vi "Send P2P FIFO to AI Loop.vi"(0 "SendDebugVal":bool, 3 "DebugVals":u32, 4 "NoOfSamples":u16, 5 "LastIterration":bool, 6 "SensorID":u8, 7 "FirstIterration":bool, 8 "ActiveLedIndex":u16, 9 "SendAiTrig":u16, 10 "SendAiCMD":u16, 11 "TimingCounter":u16) -> (1 "Trig":bool, 2 "Timed Out?":bool)   [LabVIEW 2015]
uses:
  <vilib>/rvi/eio/common/nirviEmuTemplateMethod_errors.vi
  <vilib>/eio/EIONode/EIONode.xnode
  <vilib>/rvi/DataTransferAndStorage/Container/XNode/niFpgaContainer.xnode
  <vilib>/rvi/FIFO/Fifo_Resource/nirvififoEmulationP2P.vi
  <vilib>/rvi/FIFO/Fifo_Resource/nirvififoEmulationWrite.vi
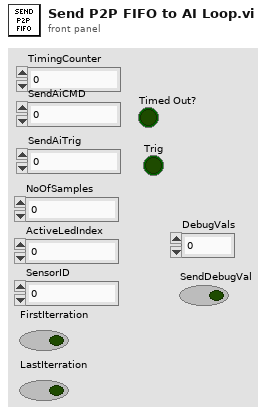
[diagram p1: front panel]
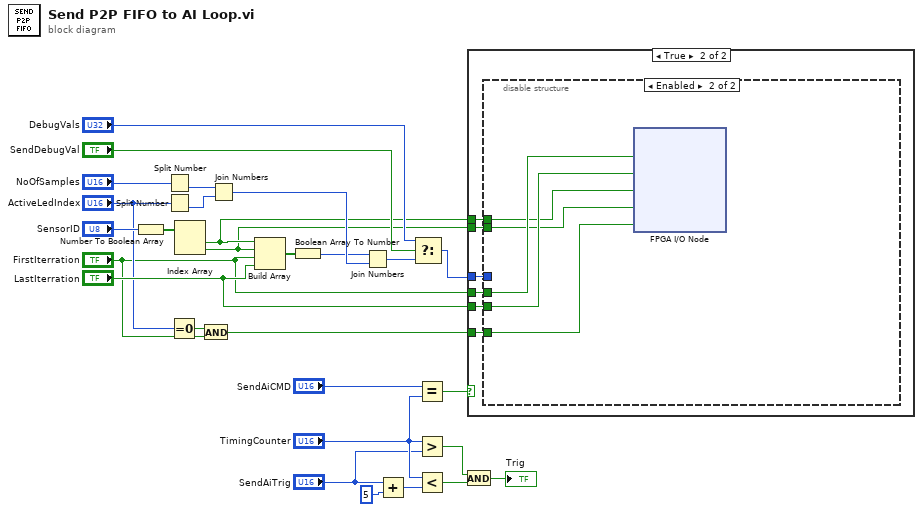
[diagram p0: block diagram]
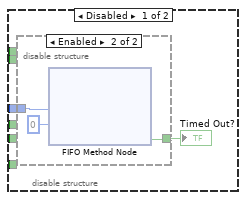
[diagram p3: hidden frame]
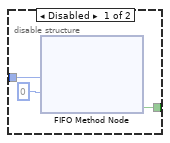
[diagram p4: hidden frame]
diagram:
  n1 = Number To Boolean Array(number="SensorID") -> (Boolean array=w15:bool[])
  n2 = Split Number(x="NoOfSamples") -> (lo(x)=w18:u8)  [unwired: 1 out]
  n3 = Split Number(x="ActiveLedIndex") -> (lo(x)=w17:u8)  [unwired: 1 out]
  n4 = Equal To 0?(x="ActiveLedIndex") -> (x = 0?=w3:bool)
  n5 = Index Array(array=w15) -> (element #1=w6:bool, element #2=w5:bool)  [unwired: 2 in]
  n6 = And(x=w3, y="FirstIterration") -> (x .and. y?=w1:bool)
  n7 = Join Numbers(hi=w18, lo=w17) -> ((hi.lo)=w14:u16)
  n8 = Build Array(w6, w5, "FirstIterration", "LastIterration") -> (w13:bool[])
  n9 = Boolean Array To Number(Boolean array=w13) -> (number=w12:u16)
  n10 = Join Numbers(hi=w12, lo=w14) -> ((hi.lo)=w11:u32)
  n11 = Add(x="SendAiTrig", y=i16 5) -> (x+y=w21:u16)
  n12 = Select(t="DebugVals", s="SendDebugVal", f=w11) -> (s? t:f=w10:u32)
  n13 = Equal?(x="SendAiCMD", y="TimingCounter") -> (x = y?=w28:bool)
  n14 = Greater?(x="TimingCounter", y="SendAiTrig") -> (0:w25:bool)
  n15 = Less?(x="TimingCounter", y=w21) -> (x < y?=w26:bool)
  n16 = And(x=w25, y=w26) -> (x .and. y?=→"Trig":bool)
  n17 = case shown="True" w28 {
    tunnel: w10 -> [_ w34]
    tunnel: "FirstIterration" -> [_ w33]
    tunnel: "LastIterration" -> [_ w32]
    tunnel: w6 -> [_ w31]
    tunnel: w5 -> [_ w30]
    tunnel: w1 -> [_ w29]
    frame False {
    }
    frame True {
      n18 = disable-structure shown="Enabled" {
        disable-tunnel: w34 -> [w36 _]
        disable-tunnel: w33 -> [_ w47]
        disable-tunnel: w32 -> [_ w46]
        disable-tunnel: w31 -> [_ w45]
        disable-tunnel: w30 -> [_ w44]
        disable-tunnel: w29 -> [_ w43]
        frame Disabled {
          n19 = disable-structure shown="Enabled" {
            disable-tunnel: w36 -> [w38 w42]
            disable-tunnel: [w37 w41] -> w35
            frame Disabled {
              n20 = xnode ("FIFO Method Node")("Element"=w38, "Timeout"=0) -> ("Timed Out?"=w37:bool)  [unwired: 1 in, 1 out]
            }
            frame Enabled {
              n21 = xnode ("FIFO Method Node")("Element"=w42, "Timeout"=0) -> ("Timed Out?"=w41:bool)  [unwired: 1 in, 1 out]
            }
          }
          "Timed Out?" <- w35
        }
        frame Enabled {
          n22 = xnode "FPGA I/O Node"("PXI_Trig2"=w47, "PXI_Trig3"=w46, "PXI_Trig4"=w45, "PXI_Trig5"=w44, "PXI_Trig6"=w43) -> ()  [unwired: 5 in, 5 out]
        }
      }
    }
  }
